vi "FindMyDensity.vi"(7 "History (s)":dbl, 10 "Cal Gas":T1) -> (1 "Density":dbl caption="Density\n(kg/m^3 = g/l)")   [LabVIEW 2016]
doc: "Calculates the density of the chosen gas at the rig conditions prevailing over the requested period.\nUses Temperature and Pressure as set by the rig's preferences.\nUse to calculate the Mass Flow Rate of gas, given a measured Volume Flow Rate."
uses:
  Anemometry Sub Vis/Controls/GasCombo.ctl
  Anemometry Sub Vis/Globals/Preference_global.vi
panel:
  out "Cal Pressure":dbl format="%#.1fmBar"
  out "Cal Temp":dbl format="%.1fC"
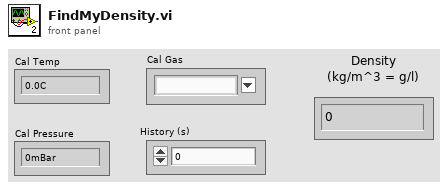
[diagram p1: front panel]
types:
  T1 = typedef "GasCombo.ctl" = string
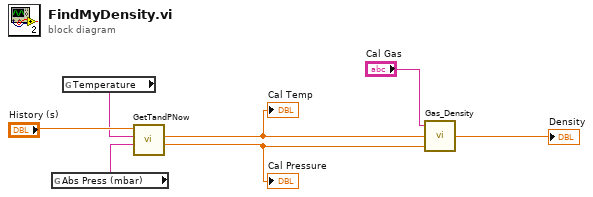
[diagram p0: block diagram]
diagram:
  n1 = global read "Preference_global.vi" "Abs Press (mbar)"() -> (w1:string)
  n2 = global read "Preference_global.vi" "Temperature"() -> (w2:string)
  n3 = call "GetTandPNow.vi"("Pressure channel"=w1, "Temperature channel"=w2, "History (s)"="History (s)") -> ("Press (mBar)"=w6:dbl, "Temp (C)"=w7:dbl)  [unwired: 7 in]
  "Cal Temp" <- w7
  "Cal Pressure" <- w6
  n4 = call "Gas_Density.vi"("Pressure (mbar)"=w6, "Temperature (C)"=w7, "Gas"="Cal Gas") -> ("Density (kg/m^3) (= g/l)"=→"Density":dbl)
